vi "meth.PrepGLue.vi"(0 "class.GLue in":refnum<class "class.GLue.lvclass">, 11 "error in":errorcluster) -> (4 "class.GLue out":refnum<class "class.GLue.lvclass">, 15 "error out":errorcluster)   [LabVIEW 2014, in "GLue.lvlib" / "class.GLue.lvclass"]
uses:
  class.GLue.lvclass
  class.GLue.lvclass/class.GLue.ctl
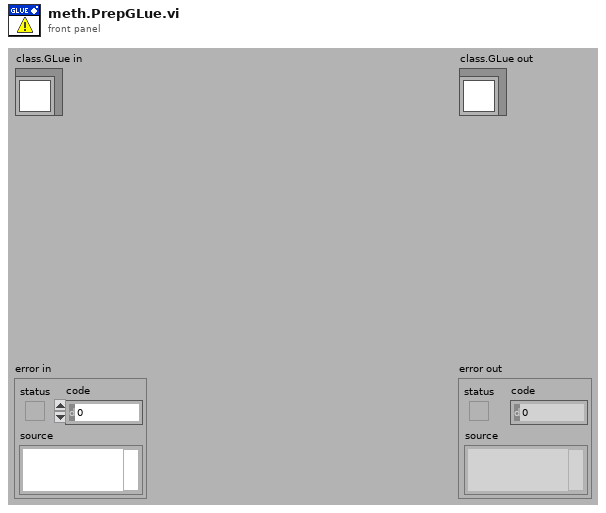
[diagram p1: front panel]
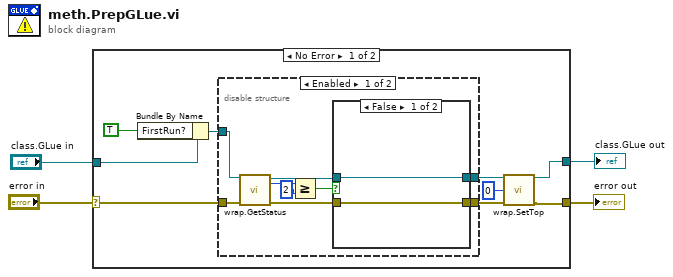
[diagram p0: block diagram]
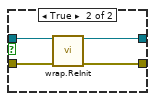
[diagram p2: hidden frame]
diagram:
  n1 = case shown="No Error" "error in" {
    selector: "error in" -> [w7 w32]
    tunnel: [w12 w32] -> w3
    tunnel: [w13 w31] -> w1
    tunnel: "class.GLue in" -> [w11 w31]
    frame No Error {
      n2 = Bundle By Name(cluster=w11, "FirstRun?"=TRUE) -> (w8:refnum<class "class.GLue.lvclass">)
      n3 = disable-structure shown="Enabled" {
        disable-tunnel: w8 -> [w22 w30]
        disable-tunnel: w7 -> [w21 w29]
        disable-tunnel: [w16 w29] -> w6
        disable-tunnel: [w14 w30] -> w5
        frame Enabled {
          n4 = call "wrap.GetStatus.vi"("class.GLue in"=w22, "error in (no error)"=w21) -> ("class.GLue out"=w15:refnum<class "class.GLue.lvclass">, "Status"=w20:i32, "error out"=w17:errorcluster)  [unwired: 11 in]
          n5 = Greater Or Equal?(x=w20, y=2) -> (x >= y?=w18:bool)
          n6 = case shown="False" w18 {
            tunnel: w17 -> [w23 w28]
            tunnel: [w23 w27] -> w16
            tunnel: w15 -> [w24 w26]
            tunnel: [w24 w25] -> w14
            frame False {
            }
            frame True {
              n7 = call "wrap.ReInit.vi"("class.GLue in"=w26, "error in (no error)"=w28) -> ("class.GLue out"=w25:refnum<class "class.GLue.lvclass">, "error out"=w27:errorcluster)  [unwired: 11 in, 1 out]
            }
          }
        }
        frame Disabled {
        }
      }
      n8 = call "wrap.SetTop.vi"("class.GLue in"=w5, "Index"=0, "error in (no error)"=w6) -> ("class.GLue out"=w13:refnum<class "class.GLue.lvclass">, "error out"=w12:errorcluster)  [unwired: 11 in]
    }
    frame Error {
    }
  }
  "error out" <- w3
  "class.GLue out" <- w1
